vi "Vision Processing.vi"(4 "error in (no error)":errorcluster, 7 "Image Size":T1=enum."320x240") -> ()   [LabVIEW 2015]
uses:
  Vision support/Camera Types.ctl
  <vilib>/Rock Robotics/WPI/Camera/WPI_CameraImageSize.ctl
  <vilib>/Rock Robotics/WPI/Camera/WPI_CameraWhite Balance Values.ctl
  <vilib>/Rock Robotics/WPI/Camera/WPI_CameraExposure Values.ctl
  <vilib>/Rock Robotics/WPI/Camera/WPI_CameraFrameRate.ctl
  Robot Global Data.vi
  <vilib>/Rock Robotics/Network Tables/NT Write Number.vi
  <vilib>/Rock Robotics/Network Tables/NT Write Numeric Array.vi
  <vilib>/vision/NI_Vision_Development_Module.lvlib
panel:
  in  "Image Size 2":T1=enum."320x240"
  out "Highest Avg Score":dbl=90.18562007395239
  in  "Min Score Threshold":i32=75
  out "Detected Targets":T2(array[cluster])=[{"Distance (ft)"=7.009585783177079, "Center"={0.0812500000000001, 0.15833333333333338}, "Normalized Rect"={"Numeric"=-0.16249999999999998, "Numeric 2"=0.30000000000000004, "Numeric 3"=0.3250000000000002, "Numeric 5"=0.01666666666666672}}] {"Normalized Rect"."Numeric 5" format="%#_2g"; "Normalized Rect"."Numeric 3" format="%#_2g"; "Normalized Rect"."Numeric 2" format="%#_2g"; "Normalized Rect"."Numeric" format="%#_2g"}
  out "Sorted Particle Scores":T3(array[cluster])=[{"Rectangle px"={"Numeric"=134.0, "Numeric 2"=84.0, "Numeric 3"=212.0, "Numeric 5"=118.0}, "Aspect Ratio"=56.61764705882355, "Area to CH"=99.3217465027554, "X"=98.71794871794873, "Y"=97.05882352941177, "Moment Factor"=83.80640246136687}] {"Moment Factor" format="%#_3g"; "Aspect Ratio" format="%#_3g"; "Area to CH" format="%#_3g"; "X" format="%#_3g"; "Y" format="%#_3g"}
  in  "Display Original":bool=TRUE
  in  "Display Mask":bool=TRUE
  out "fps":dbl=9.090909090909092
  in  "Emphasize Limit Tests":bool=TRUE
  in  "Camera Type":T4=enum."MS HD3000 square"
  in  "Aspect Fudge Factor":dbl=1.0
  in  "Score Threshold":dbl=75.0
  out "ms to process":u32=110
  out "Qualified Particles":i32=1
  in  "LED Color":T5={"Hue"={89.8844292874068, 123.8406273686592}, "Sat"={81.96428571428572, 255.0}, "Val"={27.32142857142858, 255.0}} {"Hue" scale=0.0..255.0 scale format="%#_3g"}
  out "Masked":T6(plugin-control)
  out "Original Image":T6(plugin-control)
  # "This is only the initial camera size.\nOther camera setup is done\non the diagram. Notice it is set\nonce before the loop but can be\nupdated within the loop if needed."
  # "Instructions:\nUse LED Color to threshold and build particles. Adjust calibration if needed.\nDisplays are very useful for debugging, but will slow down execution, so you\nmay want to disable once working.\nAnnotations show the rectangle and the scores from top to bottom.\nChange camera setting on diagram."
  # "Density Profile"
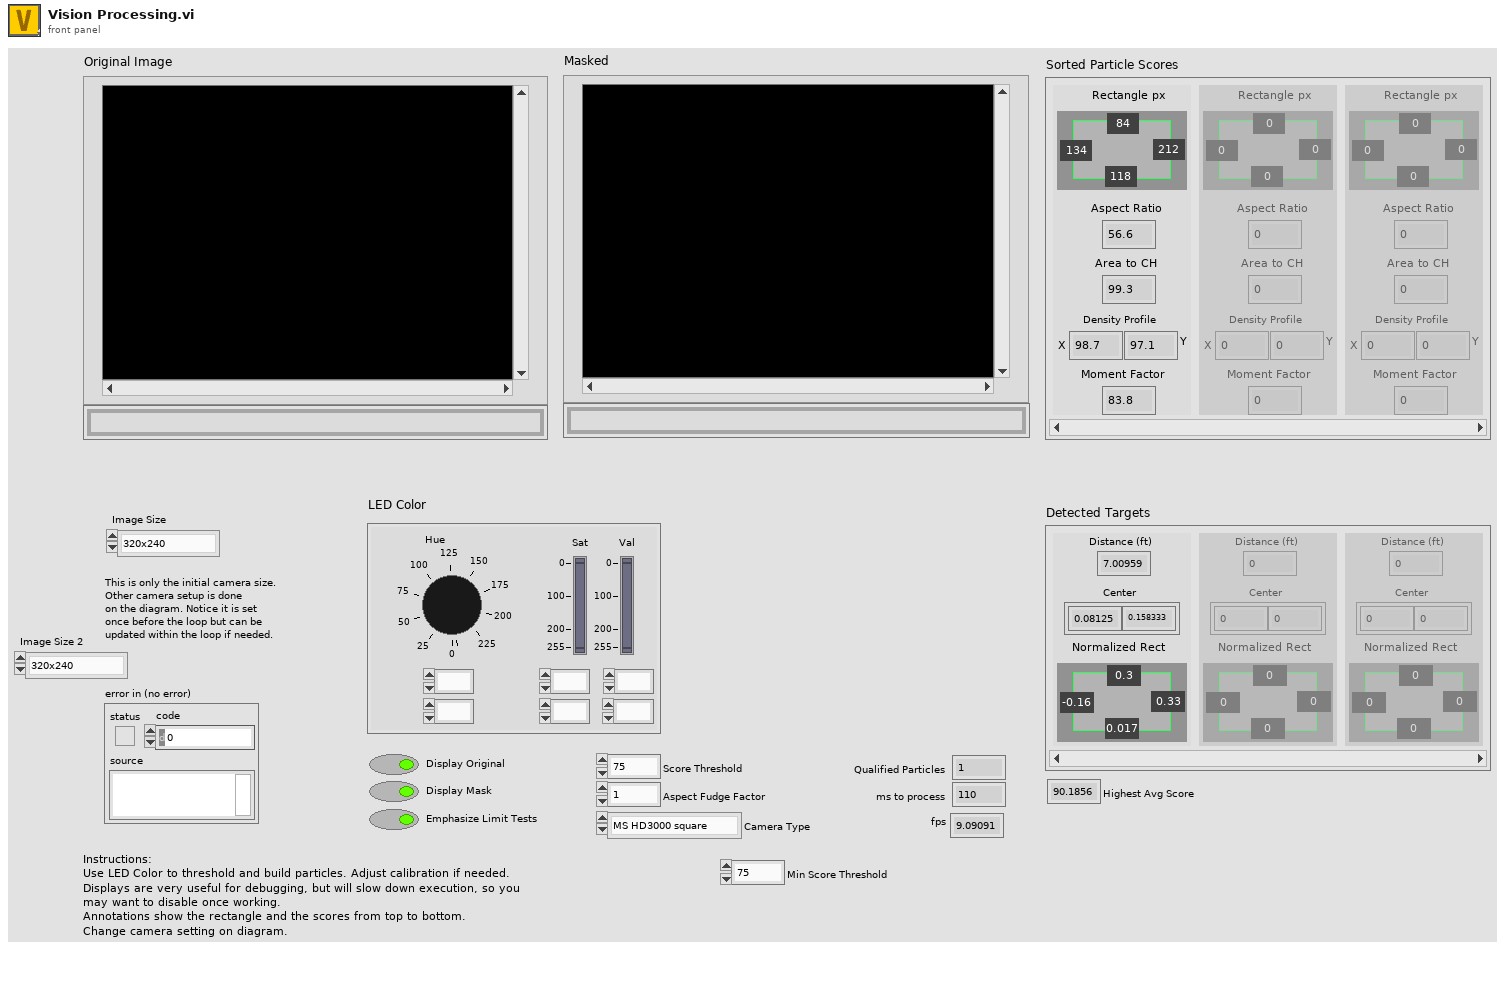
[diagram p1: front panel]
types:
  T1 = typedef "WPI_CameraImageSize.ctl" = enum16{"640x480", "320x240", "160x120", "Custom"}
  T2 = cluster{"Distance (ft)":dbl, "Center":cluster{dbl, dbl}, "Normalized Rect":cluster{"Numeric":dbl, "Numeric 2":dbl, "Numeric 3":dbl, "Numeric 5":dbl}}[]
  T3 = cluster{"Rectangle px":cluster{"Numeric":dbl, "Numeric 2":dbl, "Numeric 3":dbl, "Numeric 5":dbl}, "Aspect Ratio":dbl, "Area to CH":dbl, "X":dbl, "Y":dbl, "Moment Factor":dbl}[]
  T4 = typedef "Camera Types.ctl" = enum16{"206", "1011", "1013", "MS HD3000 square", "MS HD3000 640x480"}
  T5 = cluster{"Hue":cluster{dbl, dbl}, "Sat":cluster{dbl, dbl}, "Val":cluster{dbl, dbl}}
  T6 = typedef "IMAQ Image.ctl" = refnum<image>
  T7 = typedef "WPI_CameraFrameRate.ctl" = u32
  T8 = typedef "WPI_CameraExposure Values.ctl" = enum16{"Auto", "Flicker-free 50 Hz", "Flicker-free 60 Hz", "Hold current", "Custom"}
  T9 = typedef "WPI_CameraWhite Balance Values.ctl" = enum16{"Auto", "Fixed indoor", "Fixed outdoor 1", "Fixed outdoor 2", "Fixed fluorescent 1", "Fixed fluorescent 2", "Hold current", "Custom"}
  T10 = typedef "Particle Parameters" = i32
  T11 = typedef "Image Type" = u32
  T12 = typedef "WPI_CameraDevRef.ctl" = cluster{"Camera Address":string, "CameraStatus":errorcluster}
  T13 = cluster{"Bounding box":cluster{"left":dbl, "top":dbl, "right":dbl, "bottom":dbl}, "Aspect Ratio":dbl, "Area to CH":dbl, "X Mask":dbl, "Y Mask":dbl, "Moment":dbl}[]
  T14 = cluster{"Rectangle":cluster{"Numeric":dbl, "Numeric 2":dbl, "Numeric 3":dbl, "Numeric 5":dbl}, "L":dbl, "Area to CH":dbl, "X":dbl, "Y":dbl, "Moment Factor":dbl}[]
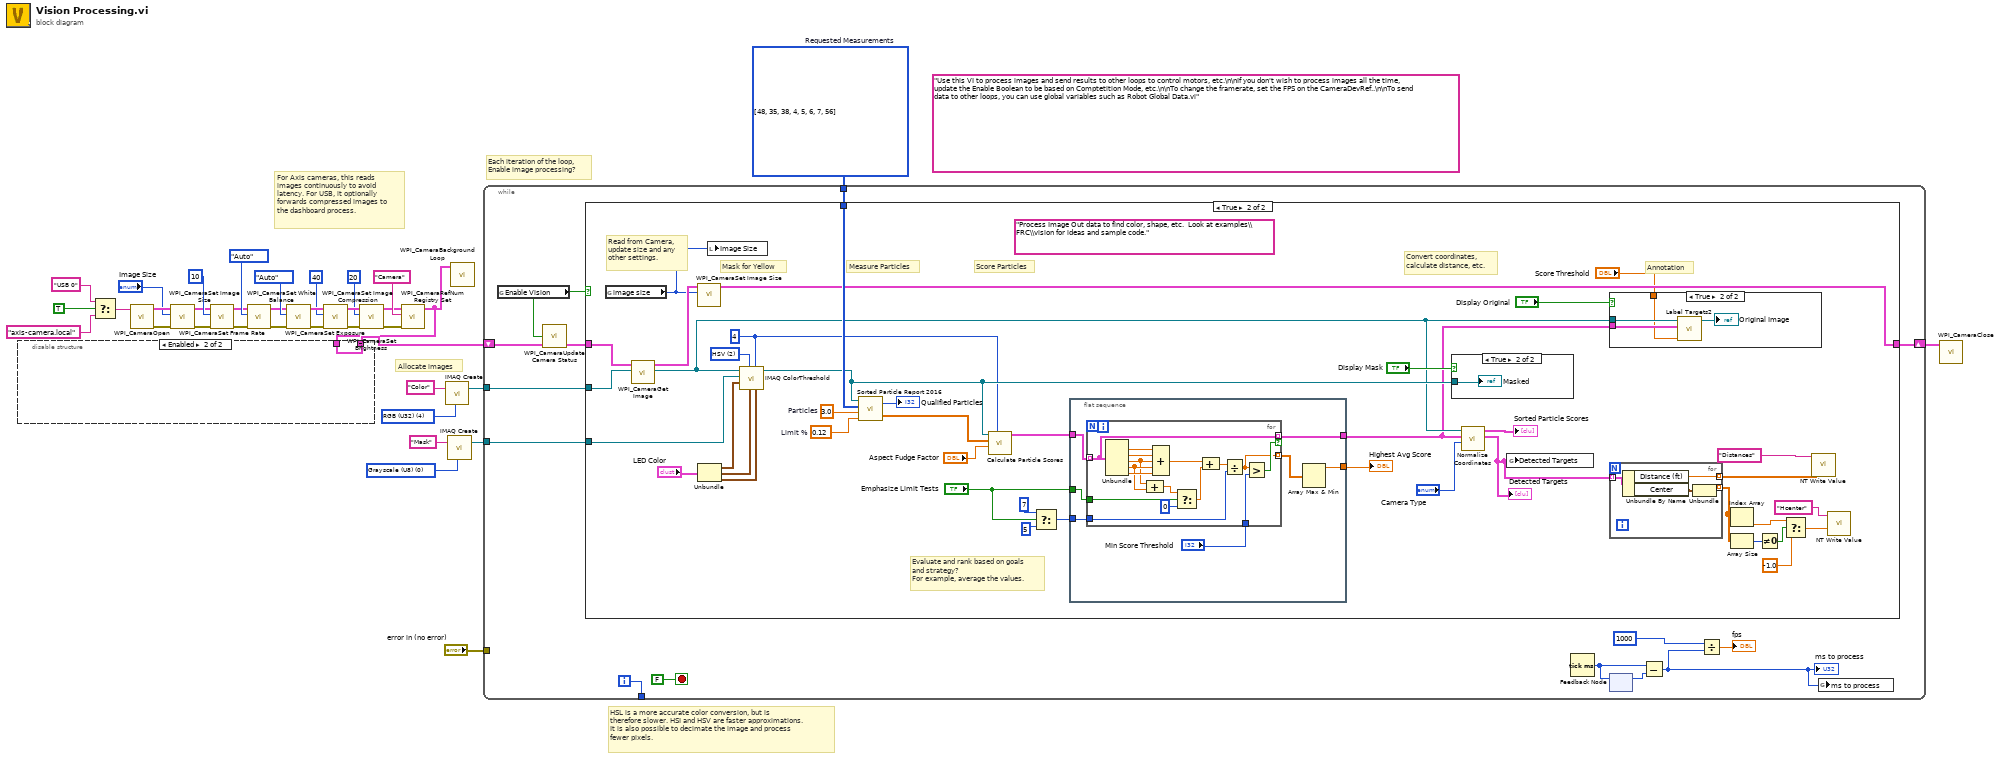
[diagram p0: block diagram]
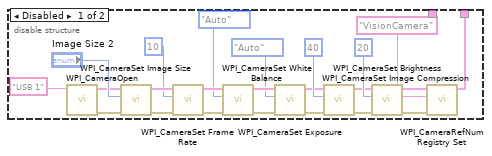
[diagram p2: hidden frame]
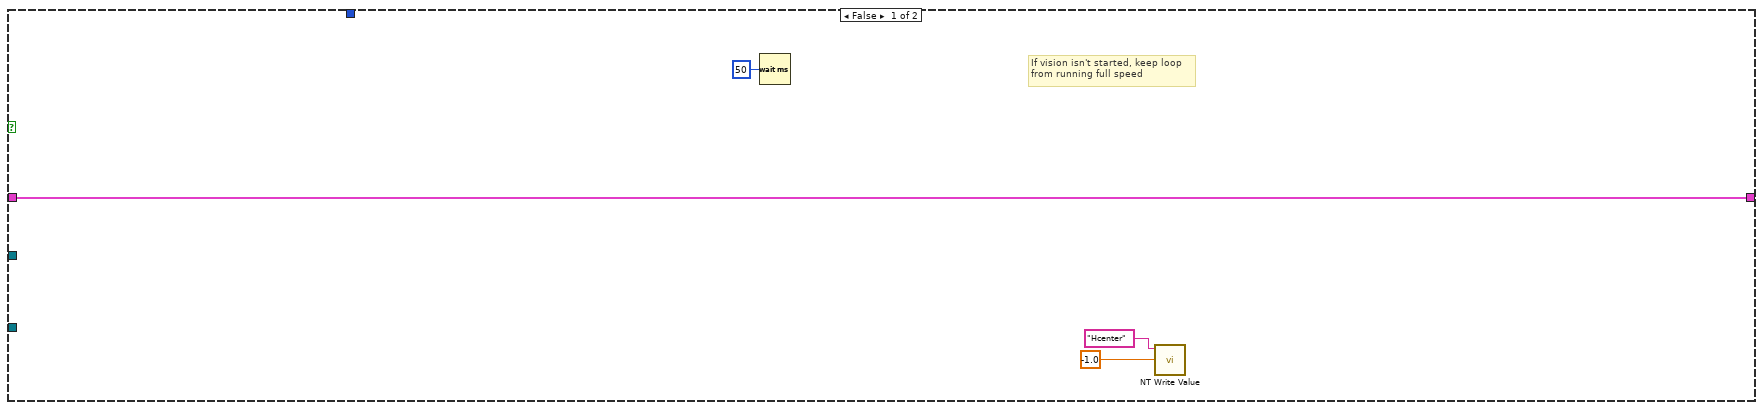
[diagram p3: hidden frame]
diagram:
  (unwired) "Use this VI to process images and send results to other loops to control motors, etc.\n\nIf you don't wish to process images all the time, update the Enable Boolean to be based on Comptetition Mode, etc.\n\nTo change the framerate, set the FPS on the CameraDevRef..\n\nTo send data to other loops, you can use global variables such as Robot Global Data.vi"
  w30 = T10[] [48, 35, 38, 4, 5, 6, 7, 56] items=["Center of Mass X", "Center of Mass Y", "First Pixel X", "First Pixel Y", "Bounding Rect Left", "Bounding Rect Top", "Bounding Rect Right", "Bounding Rect Bottom", "Max Feret Diameter Start X", "Max Feret Diameter Start Y", "Max Feret Diameter End X", "Max Feret Diameter End Y", "Max Horiz. Segment Length Left", "Max Horiz. Segment Length Right", "Max Horiz. Segment Length Row", "-", "Bounding Rect Width", "Bounding Rect Height", "Bounding Rect Diagonal", "Perimeter", "Convex Hull Perimeter", "Holes' Perimeter", "Max Feret Diameter", "Equivalent Ellipse Major Axis", "Equivalent Ellipse Minor Axis", "Equivalent Ellipse Minor Axis (Feret)", "Equivalent Rect Long Side", "Equivalent Rect Short Side", "Equivalent Rect Diagonal", "Equivalent Rect Short Side (Feret)", "Average Horiz. Segment Length", "Average Vert. Segment Length", "Hydraulic Radius", "Waddel Disk Diameter", "-", "Area", "Holes' Area", "Particle & Holes' Area", "Convex Hull Area", "Image Area", "-", "Number of Holes", "Number of Horiz. Segments", "Number of Vert. Segments", "-", "Orientation", "Max Feret Diameter Orientation", "-", "% Area/Image Area", "% Area/(Particle & Holes' Area)", "Ratio of Equivalent Ellipse Axes", "Ratio of Equivalent Rect Sides", "-", "Elongation Factor", "Compactness Factor", "Heywood Circularity Factor", "Type Factor", "-", "Sum X", "Sum Y", "Sum XX", "Sum XY", "Sum YY", "Sum XXX", "Sum XXY", "Sum XYY", "Sum YYY", "-", "Moment of Inertia XX", "Moment of Inertia XY", "Moment of Inertia YY", "Moment of Inertia XXX", "Moment of Inertia XXY", "Moment of Inertia XYY", "Moment of Inertia YYY", "Norm. Moment of Inertia XX", "Norm. Moment of Inertia XY", "Norm. Moment of Inertia YY", "Norm. Moment of Inertia XXX", "Norm. Moment of Inertia XXY", "Norm. Moment of Inertia XYY", "Norm. Moment of Inertia YYY", "Hu Moment 1", "Hu Moment 2", "Hu Moment 3", "Hu Moment 4", "Hu Moment 5", "Hu Moment 6", "Hu Moment 7"]  # Requested Measurements
  w33 = T11 0 items=["Grayscale (U8)", "Grayscale (I16)", "Grayscale (SGL)", "Complex (CSG)", "RGB (U32)", "HSL (U32)", "RGB (U64)", "Grayscale (U16)"] ("Image Type")
  w35 = T11 4 items=["Grayscale (U8)", "Grayscale (I16)", "Grayscale (SGL)", "Complex (CSG)", "RGB (U32)", "HSL (U32)", "RGB (U64)", "Grayscale (U16)"] ("Image Type")
  # "Each iteration of the loop,\nEnable image processing?"
  # "HSL is a more accurate color conversion, but is\ntherefore slower. HSI and HSV are faster approximations.\nIt is also possible to decimate the image and process\nfewer pixels."
  # "For Axis cameras, this reads\nimages continuously to avoid\nlatency. For USB, it optionally\nforwards compressed images to\nthe dashboard process."
  # "Allocate images"
  n1 = Select(t="USB 0" ("format string"), s=TRUE ("dot notation? (F)"), f="axis-camera.local" ("format string")) -> (s? t:f=w29:string)
  n2 = call <vilib>:"WPI_CameraOpen.vi"("Camera Address"=w29) -> ("error out"=w17:errorcluster, "CameraDevRef"=w16:T12)  [unwired: 1 in, 8 out]
  n3 = call <vilib>:"WPI_CameraSet Image Size.vi"("error in (no error)"=w17, "Image Size"="Image Size", "CameraDevRef"=w16) -> ("error out"=w18:errorcluster, "CameraDevRef Out"=w15:T12)  [unwired: 1 in, 6 out]
  n4 = call <vilib>:"WPI_CameraSet Frame Rate.vi"("error in (no error)"=w18, "Frame Rate (fps)"=T7 10, "CameraDevRef"=w15) -> ("error out"=w19:errorcluster, "CameraDevRef Out"=w13:T12)  [unwired: 7 out]
  n5 = call <vilib>:"WPI_CameraSet White Balance.vi"("error in (no error)"=w19, "White Balance"=WPI_CameraWhite_Balance_Values."Auto", "CameraDevRef"=w13) -> ("error out"=w20:errorcluster, "CameraDevRef Out"=w14:T12)  [unwired: 1 in, 6 out]
  n6 = call <vilib>:"WPI_CameraSet Exposure.vi"("error in (no error)"=w20, "Exposure"=WPI_CameraExposure_Values."Auto", "CameraDevRef"=w14) -> ("error out"=w21:errorcluster, "CameraDevRef Out"=w11:T12)  [unwired: 1 in, 6 out]
  n7 = call <vilib>:"WPI_CameraSet Image Compression.vi"("error in (no error)"=w21, "Compression"=40, "CameraDevRef"=w11) -> ("error out"=w22:errorcluster, "CameraDevRef Out"=w12:T12)  [unwired: 7 out]
  n8 = call <vilib>:"WPI_CameraSet Brightness.vi"("error in (no error)"=w22, "Brightness"=20, "CameraDevRef"=w12) -> ("error out"=w23:errorcluster, "CameraDevRef Out"=w3:T12)  [unwired: 7 out]
  n9 = call <vilib>:"WPI_CameraRefNum Registry Set.vi"("error in (no error)"=w23, "refnum name"="Camera", "CameraDevRef"=w3) -> ("CameraDevRef"=w1:T12)  [unwired: 1 in, 7 out]
  n10 = disable-structure shown="Enabled" {
    disable-tunnel: [w38 w60] -> w2
    disable-tunnel: w1 -> [_ w60]
    frame Disabled {
      n11 = call <vilib>:"WPI_CameraOpen.vi"("Camera Address"="USB 1" ("format string")) -> ("error out"=w48:errorcluster, "CameraDevRef"=w49:T12)  [unwired: 1 in, 8 out]
      n12 = call <vilib>:"WPI_CameraSet Image Size.vi"("error in (no error)"=w48, "Image Size"="Image Size 2", "CameraDevRef"=w49) -> ("error out"=w47:errorcluster, "CameraDevRef Out"=w50:T12)  [unwired: 1 in, 6 out]
      n13 = call <vilib>:"WPI_CameraSet Frame Rate.vi"("error in (no error)"=w47, "Frame Rate (fps)"=T7 10, "CameraDevRef"=w50) -> ("error out"=w46:errorcluster, "CameraDevRef Out"=w52:T12)  [unwired: 7 out]
      n14 = call <vilib>:"WPI_CameraSet White Balance.vi"("error in (no error)"=w46, "White Balance"=WPI_CameraWhite_Balance_Values."Auto", "CameraDevRef"=w52) -> ("error out"=w45:errorcluster, "CameraDevRef Out"=w51:T12)  [unwired: 1 in, 6 out]
      n15 = call <vilib>:"WPI_CameraSet Exposure.vi"("error in (no error)"=w45, "Exposure"=WPI_CameraExposure_Values."Auto", "CameraDevRef"=w51) -> ("error out"=w44:errorcluster, "CameraDevRef Out"=w54:T12)  [unwired: 1 in, 6 out]
      n16 = call <vilib>:"WPI_CameraSet Image Compression.vi"("error in (no error)"=w44, "Compression"=40, "CameraDevRef"=w54) -> ("error out"=w43:errorcluster, "CameraDevRef Out"=w53:T12)  [unwired: 7 out]
      n17 = call <vilib>:"WPI_CameraSet Brightness.vi"("error in (no error)"=w43, "Brightness"=20, "CameraDevRef"=w53) -> ("error out"=w42:errorcluster, "CameraDevRef Out"=w59:T12)  [unwired: 7 out]
      n18 = call <vilib>:"WPI_CameraRefNum Registry Set.vi"("error in (no error)"=w42, "refnum name"="VisionCamera", "CameraDevRef"=w59) -> ("CameraDevRef"=w38:T12)  [unwired: 1 in, 7 out]
    }
    frame Enabled {
    }
  }
  n19 = call "IMAQ Create"("Image Name"="Color", "Image Type"=w35) -> ("New Image"=w34:T6)  [unwired: 2 in, 2 out]
  n20 = call "IMAQ Create"("Image Name"="Mask", "Image Type"=w33) -> ("New Image"=w31:T6)  [unwired: 2 in, 2 out]
  n21 = call <vilib>:"WPI_CameraBackground Loop.vi"("CameraDevRef"=w1) -> ()  [unwired: 11 in]
  n22 = while {
    tunnel: w34 -> [w69]
    tunnel: w31 -> [w73]
    tunnel: w30 -> [w72]
    tunnel: "error in (no error)" -> [_]
    tunnel: [w68] -> _
    shift-right: [w64] -> w4
    shift-left: w2 -> [w66]
    i -> [w68]
    stop <- FALSE stop-if-true
    n23 = global read "Robot Global Data.vi" "Enable Vision"() -> (w67:bool)
    n24 = call <vilib>:"WPI_CameraUpdate Camera Status.vi"("CameraDevRef In"=w66, "Enable Vision"=w67) -> ("CameraDevRef Out"=w65:T12)  [unwired: 3 in]
    n25 = case shown="True" w67 {
      tunnel: w73 -> [_ w120]
      tunnel: w72 -> [_ w115]
      tunnel: w65 -> [w77 w111]
      tunnel: w69 -> [_ w110]
      tunnel: [w77 w108] -> w64
      frame False {
        # "If vision isn't started, keep loop\nfrom running full speed"
        n26 = Wait (ms)(milliseconds to wait=u32 50) -> ()  [unwired: 1 out]
        n27 = call-poly <vilib>:"NT Write Value.vi"("Numeric"=-1.0, "Name"="Hcenter") -> ()  [unwired: 9 in, 1 out]
      }
      frame True {
        w91 = 4 ("Replace Value")
        w105 = u16 2 items=["RGB", "HSL", "HSV", "HSI"] ("Color Mode")
        (unwired) "Process Image Out data to find color, shape, etc.  Look at examples\\FRC\\vision for ideas and sample code."
        w112 = 0.12  # Limit %
        w114 = 3.0  # Particles
        # "Evaluate and rank based on goals\nand strategy?\nFor example, average the values."
        # "Read from Camera,\nupdate size and any\nother settings."
        # "Measure Particles"
        # "Convert coordinates,\ncalculate distance, etc."
        # "Annotation"
        # "Score Particles"
        # "Mask for Yellow"
        n28 = global read "Robot Global Data.vi" "image size"() -> (w90:T1)
        n29 = call <vilib>:"WPI_CameraGet Image.vi"("Image"=w110, "CameraDevRef"=w111) -> ("Image Out"=w94:T6, "CameraDevRef Out"=w109:T12)  [unwired: 7 in, 1 out]
        n30 = call <vilib>:"WPI_CameraSet Image Size.vi"("Image Size"=w90, "CameraDevRef"=w109) -> ("CameraDevRef Out"=w108:T12)  [unwired: 2 in, 7 out]
        n31 = Unbundle("LED Color") -> ("Hue"=w119:cluster{dbl, dbl}, "Sat"=w118:cluster{dbl, dbl}, "Val"=w117:cluster{dbl, dbl})
        n32 = local write "Image Size"(w90) -> ()
        n33 = call "IMAQ ColorThreshold"("Blue or Luma or Val or Inten Range"=w117, "Replace Value"=w91, "Green or Sat Range"=w118, "Color Mode"=w105, "Red or Hue Range"=w119, "Image Dst"=w120, "Image Src"=w94) -> ("Image Dst Out"=w104:T6)  [unwired: 3 in, 1 out]
        n34 = call "Sorted Particle Report 2016.vi"("Min Area Size %"=w112, "Particle Count Limit"=w114, "Pixel Measurements"=w115, "Image in"=w104) -> ("Sorted Data"=w103:dbl[][], "Particles"=→"Qualified Particles":i32)
        n35 = call "Calculate Particle Scores.vi"("Pixel Value"=w91, "Aspect Fudge Factor"="Aspect Fudge Factor", "Sorted Data"=w103, "Image in"=w104) -> ("Scores"=w101:T13)  [unwired: 7 in]
        n36 = Select(t=7, s="Emphasize Limit Tests", f=5) -> (s? t:f=w98:i32)
        n37 = flat-sequence {
          tunnel: w101 -> [w135]
          tunnel: w98 -> [w133]
          tunnel: [w136] -> w97
          tunnel: [w130] -> w93
          tunnel: "Emphasize Limit Tests" -> [w134]
          frame #0 {
            n38 = for {
              tunnel: w135 -> [w150] mode=indexing
              tunnel: [w150] -> w130 mode=indexing if=w149
              tunnel: [w148] -> w131 mode=indexing
              tunnel: w133 -> [w147]
              tunnel: "Min Score Threshold" -> [w146]
              tunnel: w134 -> [w139]
              n39 = Unbundle(w150) -> ("Aspect Ratio"=w152:dbl, "Area to CH"=w151:dbl, "X Mask"=w141:dbl, "Y Mask"=w142:dbl, "Moment"=w143:dbl)  [unwired: 1 out]
              n40 = Compound Arithmetic op=ADD(w141, w142) -> (w140:dbl)
              n41 = Compound Arithmetic op=ADD(w152, w151, w141, w142, w143) -> (w145:dbl)
              n42 = Select(t=w140, s=w139, f=0) -> (s? t:f=w138:dbl)
              n43 = Compound Arithmetic op=ADD(w145, w138) -> (w144:dbl)
              n44 = Divide(x=w144, y=w147) -> (x/y=w148:dbl)
              n45 = Greater?(x=w148, y=w146) -> (0:w149:bool)
            }
            n46 = Array Max & Min(array=w131) -> (max value=w136:dbl)  [unwired: 3 out]
          }
        }
        n47 = case shown="True" "Display Mask" {
          tunnel: w104 -> [_ w129]
          frame False {
          }
          frame True {
            "Masked" <- w129
          }
        }
        n48 = call "Normalize Coordinates.vi"("Camera Type"="Camera Type", "Targets"=w93, "Image in"=w94) -> ("Found Targets"=w87:T2, "Sorted Scores"=→"Sorted Particle Scores":T14)  [unwired: 7 in]
        "Detected Targets" <- w87
        n49 = global write "Robot Global Data.vi" "Detected Targets"(w87) -> ()
        n50 = case shown="True" "Display Original" {
          tunnel: w94 -> [_ w128]
          tunnel: w93 -> [_ w126]
          tunnel: "Score Threshold" -> [_ w125]
          frame False {
          }
          frame True {
            n51 = call "Label Targets2.vi"("Score Threshold"=w125, "Targets"=w126, "Image in"=w128) -> ("Image out"=→"Original Image":T6)  [unwired: 8 in]
          }
        }
        n52 = for {
          tunnel: w87 -> [w124] mode=indexing
          tunnel: [w123] -> w86 mode=indexing
          tunnel: [w121] -> w85 mode=indexing
          n53 = Unbundle By Name(w124) -> ("Distance (ft)"=w123:dbl, "Center"=w122:cluster{dbl, dbl})
          n54 = Unbundle(w122) -> (w121:dbl)  [unwired: 1 out]
        }
        n55 = Index Array(array=w85) -> (element=w82:dbl)  [unwired: 1 in]
        n56 = Array Size(array=w85) -> (size(s)=w84:i32)
        n57 = Not Equal To 0?(x=w84) -> (x != 0?=w80:bool)
        n58 = Select(t=w82, s=w80, f=-1.0) -> (s? t:f=w81:dbl)
        n59 = call-poly <vilib>:"NT Write Value.vi"("Numeric Array"=w86, "Name"="Distances") -> ()  [unwired: 9 in, 1 out]
        n60 = call-poly <vilib>:"NT Write Value.vi"("Numeric"=w81, "Name"="Hcenter") -> ()  [unwired: 9 in, 1 out]
        "Highest Avg Score" <- w97
      }
    }
    n61 = Tick Count (ms)() -> (millisecond timer value=w70:u32)
    n62 = feedback-in #1(w70) -> ()
    n63 = feedback #1() -> (w71:u32)  [unwired: 1 in]
    n64 = Subtract(x=w70, y=w71) -> (x-y=w63:u32)
    "ms to process" <- w63
    n65 = Divide(x=1000 ("Brightness"), y=w63) -> (x/y=→"fps":dbl)
    n66 = global write "Robot Global Data.vi" "ms to process"(w63) -> ()
  }
  n67 = call <vilib>:"WPI_CameraClose.vi"("CameraDevRef"=w4) -> ()  [unwired: 1 in, 10 out]
